vi "TAT_Varient Creater.vi"(8 "error in (no error)":errorcluster) -> (0 "error out":errorcluster)   [LabVIEW 2017]
uses:
  <vilib>/Utility/miscctls.llb/LVRangeTypeDef.ctl
  <vilib>/addons/database/Connection.llb/Conn ObjectReference.ctl
  <vilib>/Utility/miscctls.llb/LVRowAndColumnUnsignedTypeDef.ctl
  b1939813-2d0c-4b6e-8ee7-2e1edd5edc28.vi
  <vilib>/Utility/config.llb/Read Key (I32).vi
  <vilib>/Utility/config.llb/Read Key (String).vi
  <vilib>/Utility/config.llb/Read Key (Boolean).vi
  <vilib>/Utility/config.llb/Write Key (U32).vi
  <vilib>/Utility/config.llb/Write Key (String).vi
  <vilib>/Utility/config.llb/Write Key (Boolean).vi
  <vilib>/Utility/config.llb/NI_LVConfig.lvlib
  <vilib>/addons/database/NI_Database_API.lvlib
panel:
  in  "HARNESS CODE":string
  in  "STATION 2\nBYPASS":bool
  in  "Vertical Slider Control":dbl(slide)=1.0 scale=1.0..-1.0
  in  "CANCLE 3":bool
  in  "PRINTING":bool
  in  "Manual print":bool
  in  "Cancle 2":bool
  in  "Delete Button":bool
  in  "Cancle":bool
  in  "Save Button":bool
  in  "TORISHI CODE":string
  in  "PART NUMBER":string
  in  "Delete Square":bool
  in  "EDIT & SAVE":bool
  out "Varient Details":string[][](table)
  in  "BATCH SIZE":u16=1 min=1 max=100 step=1
  in  "VARIENT NUMBER":u16=1 min=1 max=100 step=1
  in  "HOME":bool
  in  "UPDATE TABLE":bool
  in  "PART NAME":string(combo)
  # "Varient Creater Station 1"
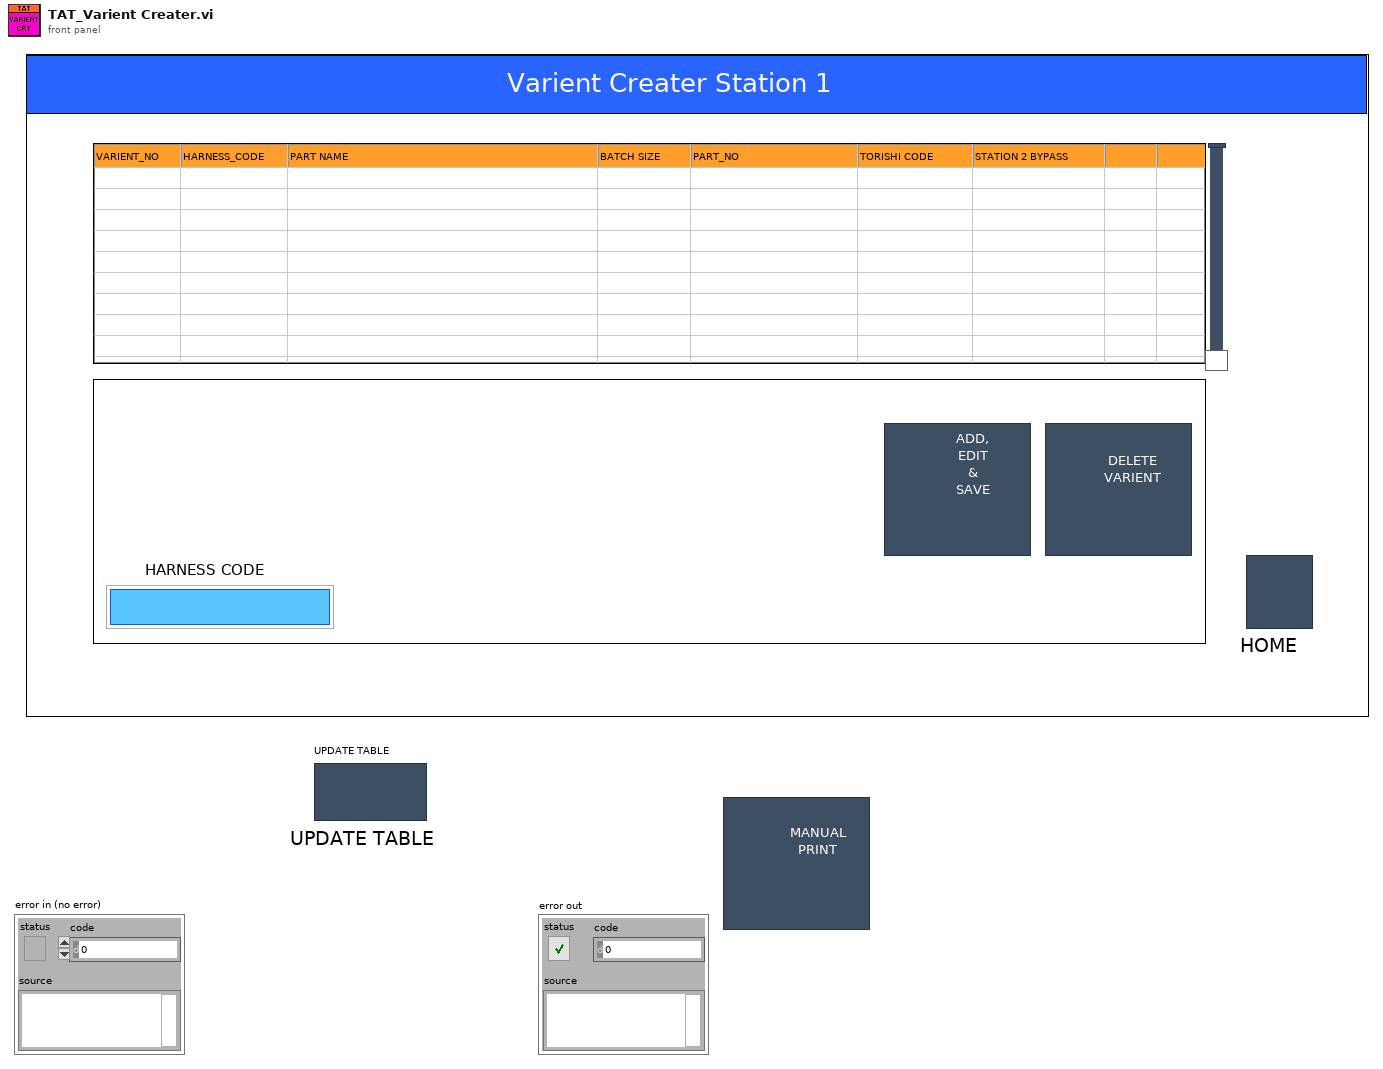
[diagram p1: front panel]
types:
  T1 = enum8{"Enabled", "Disabled", "Disabled and Grayed Out"}
  T2 = enum32{"invalid app kind", "Development System", "Run Time System", "Student Edition", "Embedded LabVIEW", "Evaluation", "Custom"}
  T3 = typedef "NI_LVConfig.lvlib/Config Data RefNum.ctl" = refnum<k1>
  T4 = typedef "LVRangeTypeDef.ctl" = cluster{"Minimum":dbl, "Maximum":dbl, "Increment":dbl, "Minor Increment":dbl, "Start":dbl}
  T5 = typedef "NI_Database_API.lvlib/Conn ObjectReference.ctl" = refnum<k1>
  T6 = cluster{"Varient number":u16, "Part name":string, "connection reference":T5, "Batch_Size":u16, "PART_NO":string, "TORISHI_CODE":string, "scanner com":refnum<visa-resource-name>, "Part Name List":string[], "Varient path":path, "Current Varient path":path, "Communication path":path, "Package path":path, "Part PRN path":path, "Station2 printer IP":string, "Station1 printer IP":string, "Current Serial Number":string, "Station1_QR":string, "Serial_Number":path, "PRIVIOUS code":string[], "Barcode station2 log":string, "Barcode station2 Up":string, "HARNESS CODE":string, "Station 1 bypass":bool}
  T7 = typedef "LVRowAndColumnUnsignedTypeDef.ctl" = cluster{"Row":u32, "Column":u32}
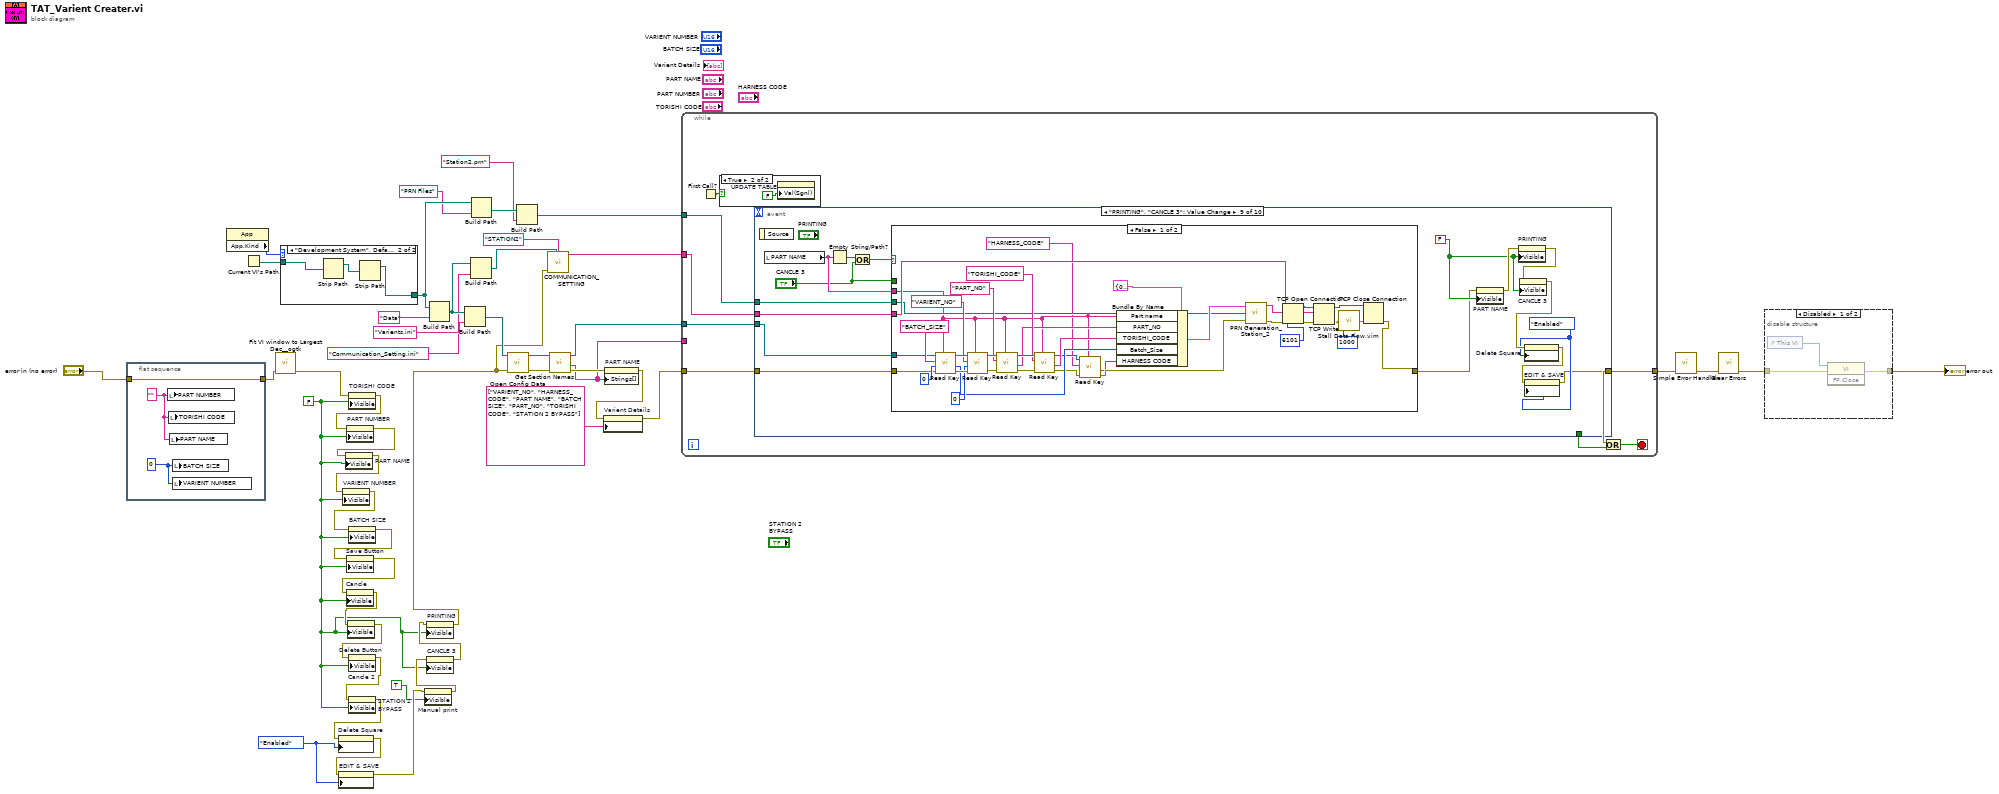
[diagram p0: block diagram]
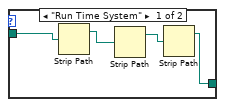
[diagram p3: hidden frame]
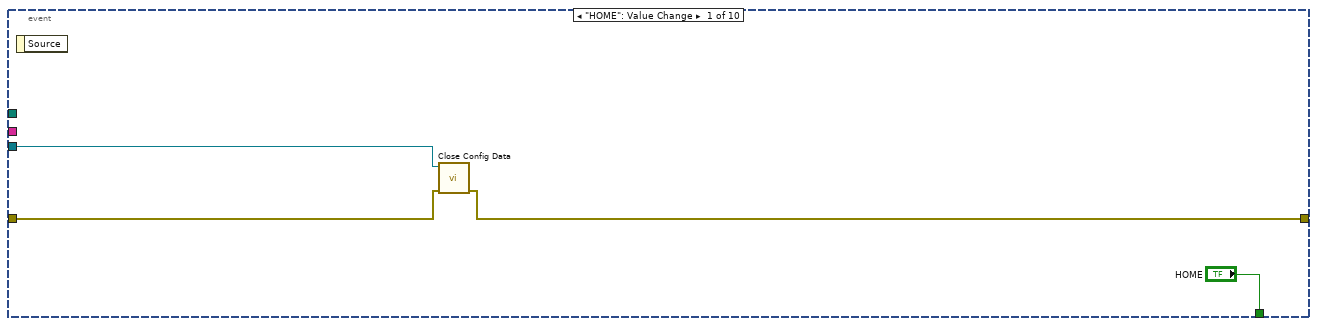
[diagram p5: hidden frame]
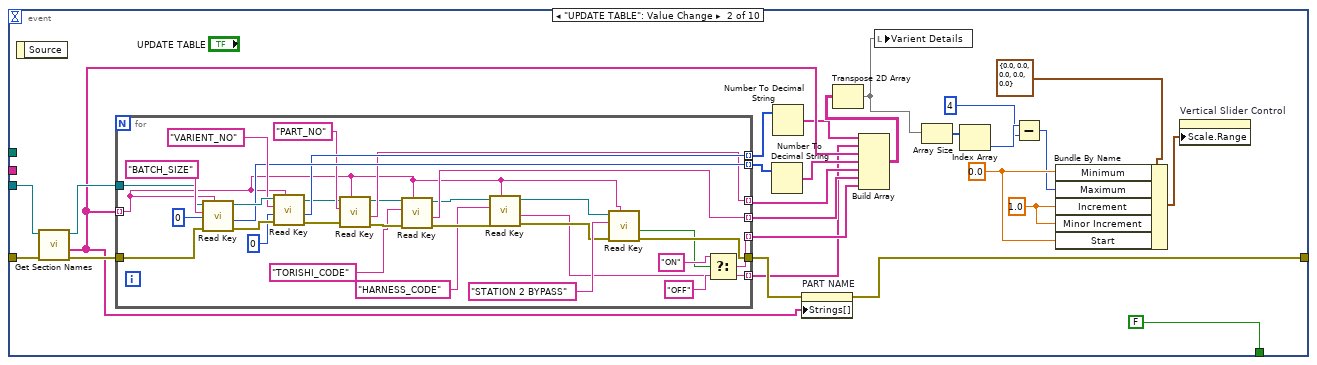
[diagram p6: hidden frame]
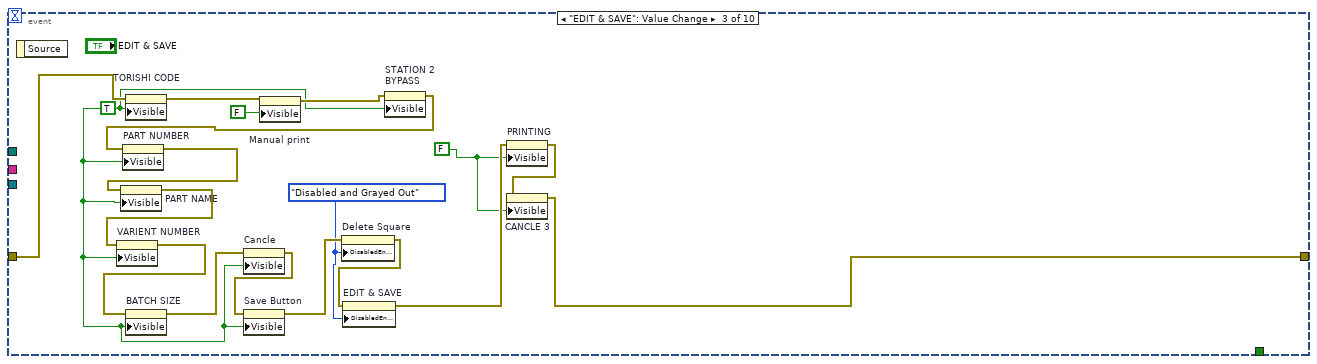
[diagram p7: hidden frame]
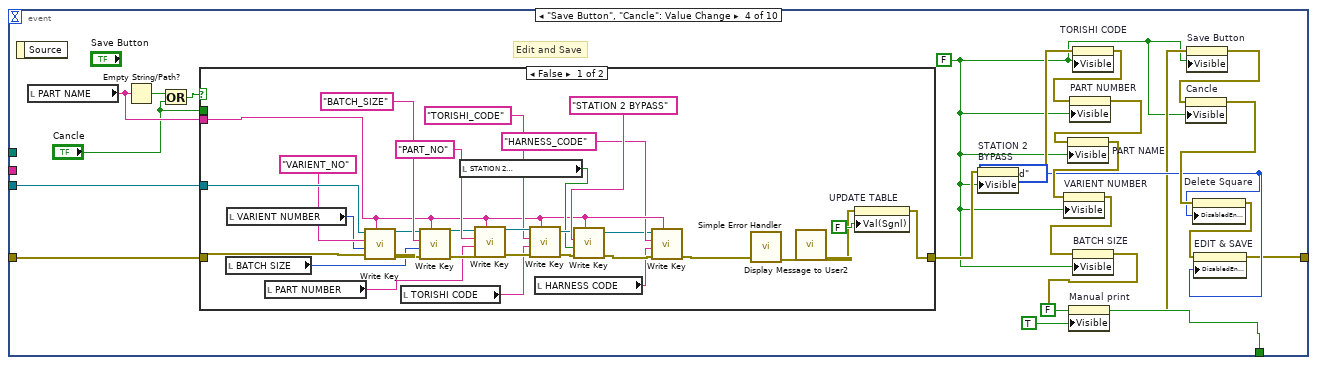
[diagram p8: hidden frame]
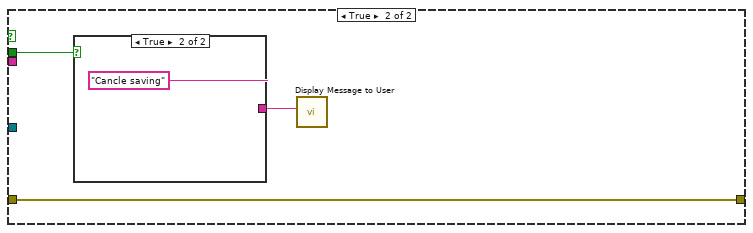
[diagram p9: hidden frame]
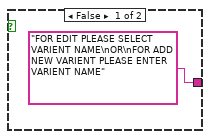
[diagram p10: hidden frame]
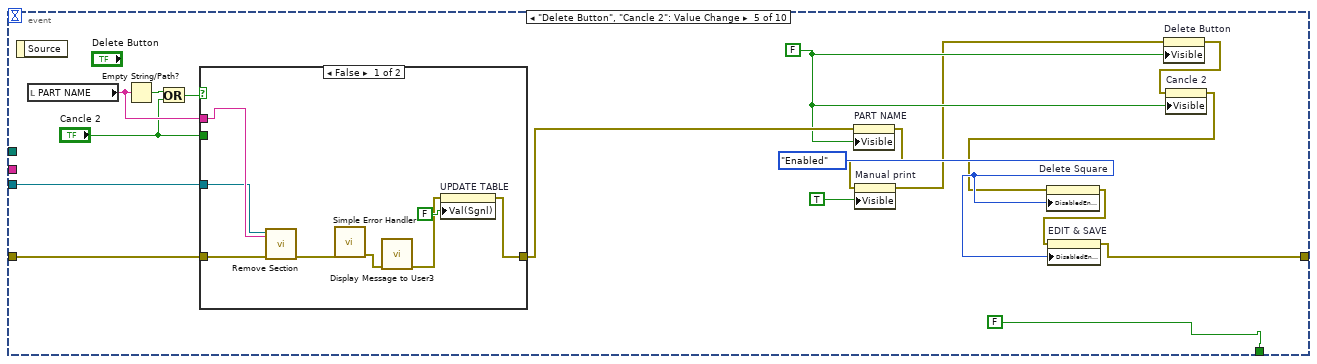
[diagram p11: hidden frame]
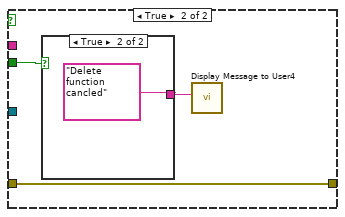
[diagram p12: hidden frame]
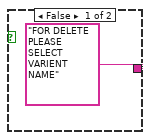
[diagram p13: hidden frame]
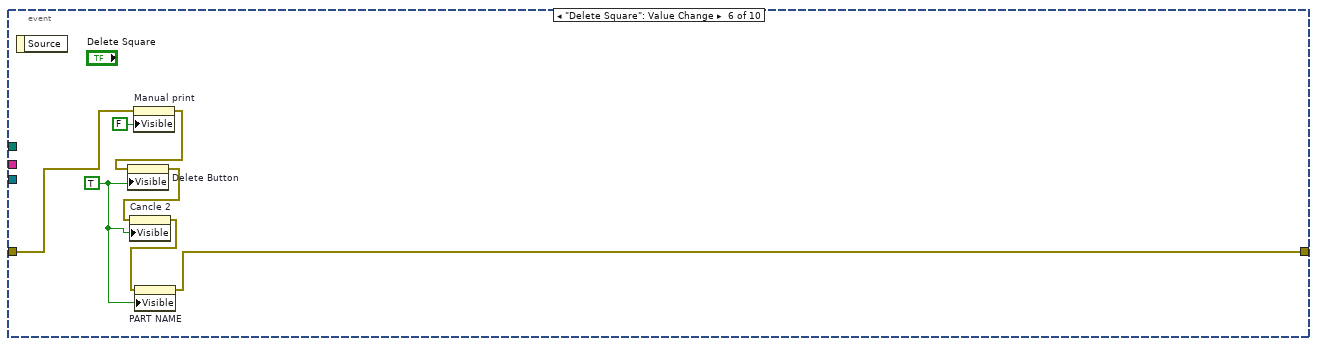
[diagram p14: hidden frame]
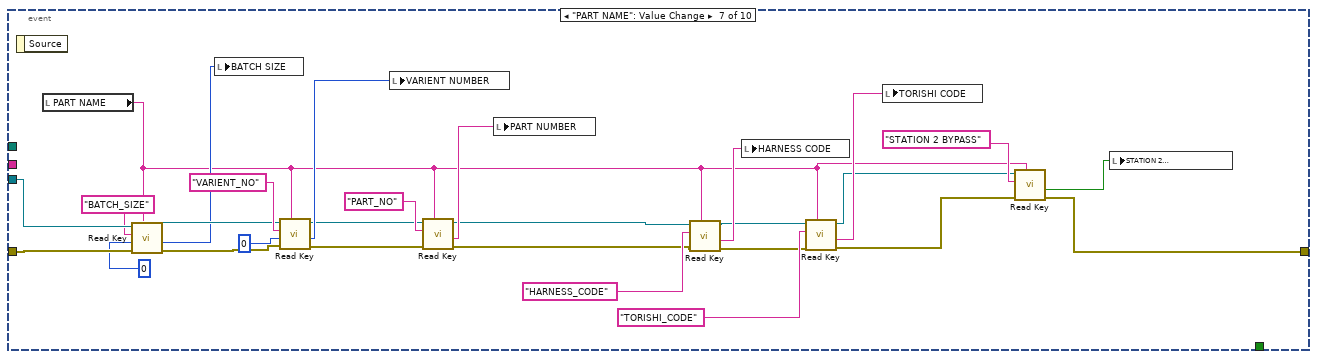
[diagram p15: hidden frame]
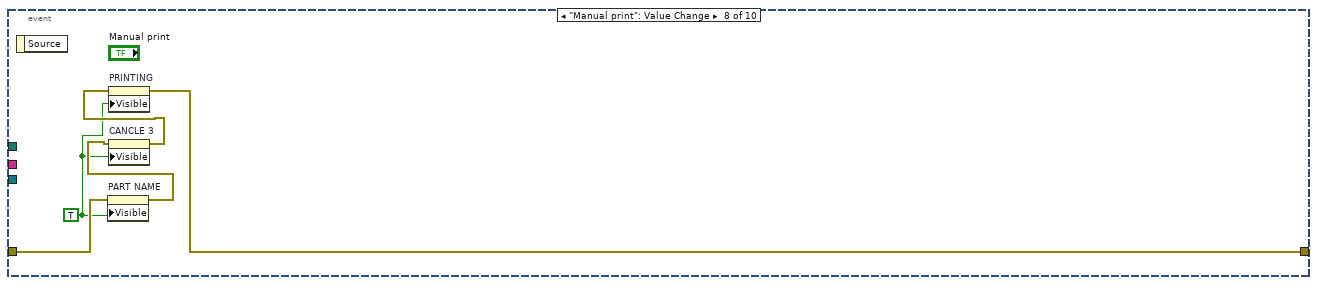
[diagram p16: hidden frame]
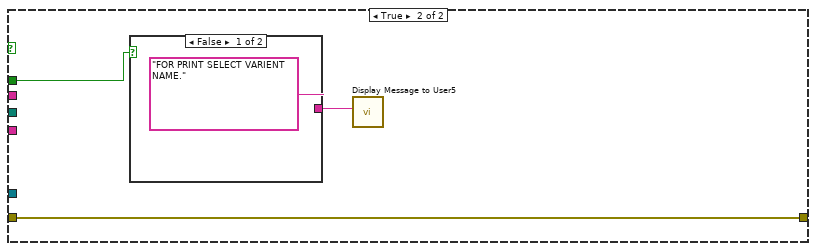
[diagram p17: hidden frame]
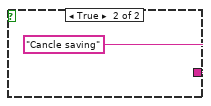
[diagram p18: hidden frame]
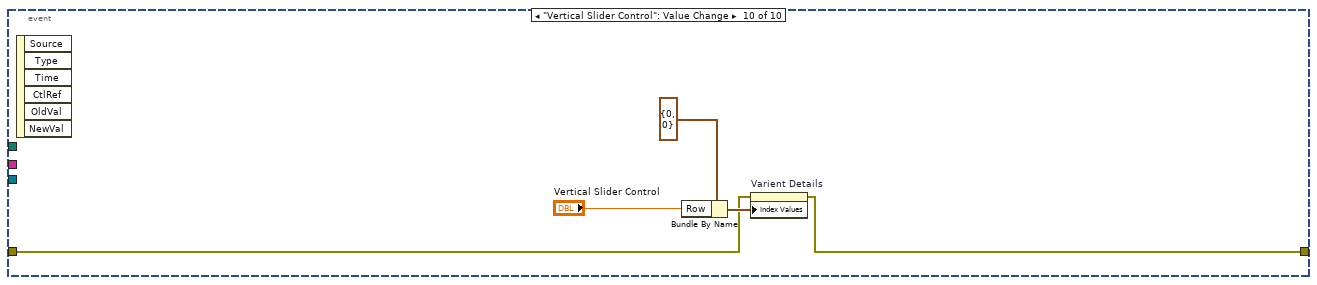
[diagram p19: hidden frame]
diagram:
  w22 = T1."Enabled" ("Disabled")
  w3 = FALSE
  n1 = flat-sequence {
    tunnel: [w49] -> w30
    tunnel: "error in (no error)" -> [w49]
    frame #0 {
      w50 = u16 0 ("BATCH SIZE")
      w51 = "" ("PART NUMBER")
      n2 = local write "PART NUMBER"(w51) -> ()
      n3 = local write "TORISHI CODE"(w51) -> ()
      n4 = local write "PART NAME"(w51) -> ()
      n5 = local write "BATCH SIZE"(w50) -> ()
      n6 = local write "VARIENT NUMBER"(w50) -> ()
    }
  }
  n7 = property class="App"() -> ("App.Kind"=w43:T2)  [unwired: 2 in, 2 out]
  n8 = Current VI's Path() -> (path=w44:path)
  n9 = call <userlib>:"Fit VI window to Largest Dec__ogtk.vi"("error in (no error)"=w30) -> ("error out"=w25:errorcluster)  [unwired: 5 in, 1 out]
  n10 = case shown="\"Development System\", Default" w43 {
    tunnel: w44 -> [w53 w57]
    tunnel: [w52 w56] -> w8
    frame "Run Time System" {
      n11 = Strip Path(path=w53) -> (stripped path=w55:path)  [unwired: 1 out]
      n12 = Strip Path(path=w55) -> (stripped path=w54:path)  [unwired: 1 out]
      n13 = Strip Path(path=w54) -> (stripped path=w52:path)  [unwired: 1 out]
    }
    frame "Development System", Default {
      n14 = Strip Path(path=w57) -> (stripped path=w58:path)  [unwired: 1 out]
      n15 = Strip Path(path=w58) -> (stripped path=w56:path)  [unwired: 1 out]
    }
  }
  n16 = property on="TORISHI CODE" class="Str"(error in=w25, "Visible"=w3) -> (error out=w29:errorcluster)  [unwired: 1 in, 1 out]
  n17 = property on="PART NUMBER" class="Str"(error in=w29, "Visible"=w3) -> (error out=w28:errorcluster)  [unwired: 1 in, 1 out]
  n18 = property on="PART NAME" class="CmbBox"(error in=w28, "Visible"=w3) -> (error out=w27:errorcluster)  [unwired: 1 in, 1 out]
  n19 = property on="VARIENT NUMBER" class="DigNum (strict)"(error in=w27, "Visible"=w3) -> (error out=w26:errorcluster)  [unwired: 1 in, 1 out]
  n20 = property on="BATCH SIZE" class="DigNum (strict)"(error in=w26, "Visible"=w3) -> (error out=w24:errorcluster)  [unwired: 1 in, 1 out]
  n21 = property on="Save Button" class="Bool"(error in=w24, "Visible"=w3) -> (error out=w21:errorcluster)  [unwired: 1 in, 1 out]
  n22 = property on="Cancle" class="Bool"(error in=w21, "Visible"=w3) -> (error out=w20:errorcluster)  [unwired: 1 in, 1 out]
  n23 = property on="Delete Button" class="Bool"(error in=w20, "Visible"=w3) -> (error out=w19:errorcluster)  [unwired: 1 in, 1 out]
  n24 = property on="Cancle 2" class="Bool"(error in=w19, "Visible"=w3) -> (error out=w2:errorcluster)  [unwired: 1 in, 1 out]
  n25 = property on="STATION 2\nBYPASS" class="Bool (strict)"(error in=w2, "Visible"=w3) -> (error out=w1:errorcluster)  [unwired: 1 in, 1 out]
  n26 = property on="Delete Square" class="Bool"(error in=w1, "DisabledEnum"=w22) -> (error out=w23:errorcluster)  [unwired: 1 in, 1 out]
  n27 = property on="EDIT & SAVE" class="Bool"(error in=w23, "DisabledEnum"=w22) -> (error out=w17:errorcluster)  [unwired: 1 in, 1 out]
  n28 = property on="Manual print" class="Bool"(error in=w17, "Visible"=TRUE) -> (error out=w16:errorcluster)  [unwired: 1 in, 1 out]
  n29 = property on="CANCLE 3" class="Bool"(error in=w16, "Visible"=w3) -> (error out=w18:errorcluster)  [unwired: 1 in, 1 out]
  n30 = property on="PRINTING" class="Bool"(error in=w18, "Visible"=w3) -> (error out=w10:errorcluster)  [unwired: 1 in, 1 out]
  n31 = Build Path(base path=w8, name or relative path="Data") -> (appended path=w14:path)
  n32 = Build Path(base path=w14, name or relative path="Varients.ini") -> (appended path=w42:path)
  n33 = Build Path(base path=w14, name or relative path="Communication_Setting.ini") -> (appended path=w11:path)
  n34 = Build Path(base path=w8, name or relative path="PRN Files") -> (appended path=w6:path)
  n35 = call <vilib>:"Open Config Data.vi"("error in (no error)"=w10, "configuration file path"=w42) -> ("error out"=w38:errorcluster, "refnum"=w39:T3)  [unwired: 7 in, 1 out]
  n36 = Build Path(base path=w6, name or relative path="Station2.prn") -> (appended path=w4:path)
  n37 = call "COMMUNICATION_SETTING.vi"("communication path"=w11, "error in"=w10, "STATION"="STATION2") -> ("PRINT_COM"=w9:string)  [unwired: 6 in, 2 out]
  n38 = call <vilib>:"Get Section Names.vi"("error in (no error)"=w38, "refnum"=w39) -> ("error out"=w37:errorcluster, "section names"=w32:string[], "refnum out"=w36:T3)  [unwired: 7 in]
  n39 = property on="PART NAME" class="CmbBox"(error in=w37, "Strings[]"=w32) -> (error out=w35:errorcluster)  [unwired: 1 in, 1 out]
  n40 = property on="Varient Details" class="Tbl (strict)"(error in=w35, "Column Headers[]"=string[] ["VARIENT_NO", "HARNESS_CODE", "PART NAME", "BATCH SIZE", "PART_NO", "TORISHI CODE", "STATION 2 BYPASS"] ("Column Header Strings[]")) -> (error out=w34:errorcluster)  [unwired: 1 in, 1 out]
  n41 = while {
    tunnel: w34 -> [w65]
    tunnel: [w63] -> w45
    tunnel: w36 -> [w62]
    tunnel: w32 -> [_]
    tunnel: w9 -> [w60]
    tunnel: w4 -> [w59]
    stop <- w64 stop-if-true
    n42 = First Call?() -> (First Call?: T/F=w61:bool)
    n43 = case shown="True" w61 {
      frame False {
      }
      frame True {
        n44 = property on="UPDATE TABLE" class="Bool (strict)"("Val(Sgnl)"=FALSE) -> ()  [unwired: 2 in, 2 out]
      }
    }
    n45 = event shown="[8] \"PRINTING\", \"CANCLE 3\": Value Change" {
      selector: _ -> [_ _ _ _ _ _ _ _ _ _]
      dyn-events: _ -> [_ _ _ _ _ _ _ _ _ _]
      timeout: _ -> [_ _ _ _ _ _ _ _ _ _]
      tunnel: ["HOME" FALSE ("stop") _ FALSE ("stop") FALSE ("stop") _ _ _ _ _] -> w66
      tunnel: w65 -> [w70 w92 w143 w166 w218 w235 w268 w271 w289 w332]
      tunnel: [w69 w84 w133 w153 w210 w238 w251 w270 w278 w333] -> w63
      tunnel: w62 -> [w68 w90 _ w167 w219 _ w267 _ w285 _]
      tunnel: w60 -> [_ _ _ _ _ _ _ _ w276 _]
      tunnel: w59 -> [_ _ _ _ _ _ _ _ w275 _]
      event "HOME": Value Change {
        n46 = event-data() -> ()  [unwired: 1 in, 1 out]
        n47 = call <vilib>:"Close Config Data.vi"("error in (no error)"=w70, "refnum"=w68) -> ("error out"=w69:errorcluster)  [unwired: 8 in, 1 out]
      }
      event "UPDATE TABLE": Value Change {
        w81 = 1.0 ("Increment")
        w80 = 0.0 ("Minimum")
        n48 = event-data() -> ()  [unwired: 1 in, 1 out]
        n49 = call <vilib>:"Get Section Names.vi"("error in (no error)"=w92, "refnum"=w90) -> ("error out"=w91:errorcluster, "section names"=w85:string[], "refnum out"=w89:T3)  [unwired: 7 in]
        n50 = for {
          tunnel: [w110] -> w86
          tunnel: w91 -> [w122]
          tunnel: w85 -> [w102] mode=indexing
          tunnel: w89 -> [w121]
          tunnel: [w120] -> w95 mode=indexing
          tunnel: [w119] -> w96 mode=indexing
          tunnel: [w115] -> w88 mode=indexing
          tunnel: [w111] -> w87 mode=indexing
          tunnel: [w105] -> w74 mode=indexing
          tunnel: [w98] -> w72 mode=indexing
          n51 = call-poly <vilib>:"Read Key.vi"("section"=w102, "error in (no error)"=w122, "default value"=0, "key"="BATCH_SIZE", "refnum"=w121) -> ("error out"=w128:errorcluster, "value"=w120:i32, "refnum out"=w127:T3)  [unwired: 3 in, 1 out]
          n52 = call-poly <vilib>:"Read Key.vi"("section"=w102, "error in (no error)"=w128, "default value"=0, "key"="VARIENT_NO", "refnum"=w127) -> ("error out"=w118:errorcluster, "value"=w119:i32, "refnum out"=w116:T3)  [unwired: 3 in, 1 out]
          n53 = call-poly <vilib>:"Read Key.vi"("section"=w102, "error in (no error)"=w118, "key"="PART_NO", "refnum"=w116) -> ("error out"=w114:errorcluster, "value"=w115:string, "refnum out"=w113:T3)  [unwired: 4 in, 1 out]
          n54 = call-poly <vilib>:"Read Key.vi"("section"=w102, "error in (no error)"=w114, "key"="TORISHI_CODE", "refnum"=w113) -> ("error out"=w101:errorcluster, "value"=w111:string, "refnum out"=w104:T3)  [unwired: 4 in, 1 out]
          n55 = call-poly <vilib>:"Read Key.vi"("section"=w102, "error in (no error)"=w101, "key"="HARNESS_CODE", "refnum"=w104) -> ("error out"=w100:errorcluster, "value"=w98:string, "refnum out"=w103:T3)  [unwired: 4 in, 1 out]
          n56 = call-poly <vilib>:"Read Key.vi"("section"=w102, "error in (no error)"=w100, "key"="STATION 2 BYPASS", "refnum"=w103) -> ("error out"=w110:errorcluster, "value"=w106:bool)  [unwired: 4 in, 2 out]
          n57 = Select(t="ON" ("String"), s=w106, f="OFF" ("String")) -> (s? t:f=w105:string)
        }
        n58 = Number To Decimal String(number=w95) -> (decimal integer string=w94:string[])  [unwired: 1 in]
        n59 = Number To Decimal String(number=w96) -> (decimal integer string=w73:string[])  [unwired: 1 in]
        n60 = property on="PART NAME" class="CmbBox"(error in=w86, "Strings[]"=w85) -> (error out=w84:errorcluster)  [unwired: 1 in, 1 out]
        n61 = Build Array(w73, w72, w85, w94, w88, w87, w74) -> (w93:string[][])
        n62 = Transpose 2D Array(2D array=w93) -> (transposed array=w83:string[][])
        n63 = local write "Varient Details"(w83) -> ()
        n64 = Array Size(array=w83) -> (size(s)=w82:i32[])
        n65 = Index Array(array=w82) -> (element=w77:i32)  [unwired: 1 in]
        n66 = Subtract(x=w77, y=4) -> (x-y=w76:i32)
        n67 = Bundle By Name(cluster=T4 {"Minimum"=0.0, "Maximum"=0.0, "Increment"=0.0, "Minor Increment"=0.0, "Start"=0.0} ("Scale.Range"), "Minimum"=w80, "Maximum"=w76, "Increment"=w81, "Minor Increment"=w81, "Start"=w80) -> (w79:T4)
        n68 = property on="Vertical Slider Control" class="Slide (strict)"("Scale.Range"=w79) -> ()  [unwired: 2 in, 2 out]
      }
      event "EDIT & SAVE": Value Change {
        w132 = FALSE
        w140 = T1."Disabled and Grayed Out" ("Disabled")
        w129 = TRUE
        n69 = event-data() -> ()  [unwired: 1 in, 1 out]
        n70 = property on="TORISHI CODE" class="Str"(error in=w143, "Visible"=w129) -> (error out=w137:errorcluster)  [unwired: 1 in, 1 out]
        n71 = property on="Manual print" class="Bool"(error in=w137, "Visible"=FALSE) -> (error out=w131:errorcluster)  [unwired: 1 in, 1 out]
        n72 = property on="STATION 2\nBYPASS" class="Bool (strict)"(error in=w131, "Visible"=w129) -> (error out=w130:errorcluster)  [unwired: 1 in, 1 out]
        n73 = property on="PART NUMBER" class="Str"(error in=w130, "Visible"=w129) -> (error out=w144:errorcluster)  [unwired: 1 in, 1 out]
        n74 = property on="PART NAME" class="CmbBox"(error in=w144, "Visible"=w129) -> (error out=w145:errorcluster)  [unwired: 1 in, 1 out]
        n75 = property on="VARIENT NUMBER" class="DigNum (strict)"(error in=w145, "Visible"=w129) -> (error out=w146:errorcluster)  [unwired: 1 in, 1 out]
        n76 = property on="BATCH SIZE" class="DigNum (strict)"(error in=w146, "Visible"=w129) -> (error out=w138:errorcluster)  [unwired: 1 in, 1 out]
        n77 = property on="Cancle" class="Bool"(error in=w138, "Visible"=w129) -> (error out=w139:errorcluster)  [unwired: 1 in, 1 out]
        n78 = property on="Save Button" class="Bool"(error in=w139, "Visible"=w129) -> (error out=w142:errorcluster)  [unwired: 1 in, 1 out]
        n79 = property on="Delete Square" class="Bool"(error in=w142, "DisabledEnum"=w140) -> (error out=w141:errorcluster)  [unwired: 1 in, 1 out]
        n80 = property on="EDIT & SAVE" class="Bool"(error in=w141, "DisabledEnum"=w140) -> (error out=w134:errorcluster)  [unwired: 1 in, 1 out]
        n81 = property on="PRINTING" class="Bool"(error in=w134, "Visible"=w132) -> (error out=w135:errorcluster)  [unwired: 1 in, 1 out]
        n82 = property on="CANCLE 3" class="Bool"(error in=w135, "Visible"=w132) -> (error out=w133:errorcluster)  [unwired: 1 in, 1 out]
      }
      event "Save Button", "Cancle": Value Change {
        w154 = T1."Enabled" ("Disabled")
        w147 = FALSE
        # "Edit and Save"
        n83 = event-data() -> ()  [unwired: 1 in, 1 out]
        n84 = local read "PART NAME"() -> (w165:string)
        n85 = Empty String/Path?(string/path=w165) -> (empty?=w164:bool)
        n86 = Or(x=w164, y="Cancle") -> (x .or. y?=w163:bool)
        n87 = case shown="False" w163 {
          tunnel: w166 -> [w197 w201]
          tunnel: [w191 w201] -> w149
          tunnel: w167 -> [w195 _]
          tunnel: w165 -> [w174 _]
          tunnel: "Cancle" -> [_ w199]
          frame False {
            n88 = local read "BATCH SIZE"() -> (w190:u16)
            n89 = local read "VARIENT NUMBER"() -> (w189:u16)
            n90 = local read "PART NUMBER"() -> (w179:string)
            n91 = call-poly <vilib>:"Write Key.vi"("section"=w174, "error in (no error)"=w197, "value"=w189, "key"="VARIENT_NO", "refnum"=w195) -> ("error out"=w196:errorcluster, "refnum out"=w194:T3)  [unwired: 4 in, 1 out]
            n92 = local read "TORISHI CODE"() -> (w180:string)
            n93 = call-poly <vilib>:"Write Key.vi"("section"=w174, "error in (no error)"=w196, "value"=w190, "key"="BATCH_SIZE", "refnum"=w194) -> ("error out"=w184:errorcluster, "refnum out"=w182:T3)  [unwired: 4 in, 1 out]
            n94 = local read "STATION 2\nBYPASS"() -> (w175:bool)
            n95 = call-poly <vilib>:"Write Key.vi"("section"=w174, "error in (no error)"=w184, "value"=w179, "key"="PART_NO", "refnum"=w182) -> ("error out"=w185:errorcluster, "refnum out"=w186:T3)  [unwired: 4 in, 1 out]
            n96 = call-poly <vilib>:"Write Key.vi"("section"=w174, "error in (no error)"=w185, "value"=w180, "key"="TORISHI_CODE", "refnum"=w186) -> ("error out"=w177:errorcluster, "refnum out"=w176:T3)  [unwired: 4 in, 1 out]
            n97 = local read "HARNESS CODE"() -> (w169:string)
            n98 = call-poly <vilib>:"Write Key.vi"("section"=w174, "error in (no error)"=w177, "value"=w175, "key"="STATION 2 BYPASS", "refnum"=w176) -> ("error out"=w173:errorcluster, "refnum out"=w170:T3)  [unwired: 4 in, 1 out]
            n99 = call-poly <vilib>:"Write Key.vi"("section"=w174, "error in (no error)"=w173, "value"=w169, "key"="HARNESS_CODE", "refnum"=w170) -> ("error out"=w172:errorcluster)  [unwired: 4 in, 2 out]
            n100 = call <vilib>:"Simple Error Handler.vi"("error in (no error)"=w172) -> ("error out"=w188:errorcluster)  [unwired: 4 in, 4 out]
            n101 = call "Display Message to User2"("error in (no error)"=w188) -> ("error out"=w187:errorcluster)  [unwired: 9 in, 1 out]
            n102 = property on="UPDATE TABLE" class="Bool (strict)"(error in=w187, "Val(Sgnl)"=FALSE) -> (error out=w191:errorcluster)  [unwired: 1 in, 1 out]
          }
          frame True {
            n103 = case shown="True" w199 {
              tunnel: ["FOR EDIT PLEASE SELECT VARIENT NAME\nOR\nFOR ADD NEW VARIENT PLEASE ENTER VARIENT NAME" "Cancle saving"] -> w200
              frame False {
              }
              frame True {
              }
            }
            n104 = call "Display Message to User"("Message"=w200) -> ()  [unwired: 9 in, 2 out]
          }
        }
        n105 = property on="STATION 2\nBYPASS" class="Bool (strict)"(error in=w149, "Visible"=w147) -> (error out=w148:errorcluster)  [unwired: 1 in, 1 out]
        n106 = property on="TORISHI CODE" class="Str"(error in=w148, "Visible"=w147) -> (error out=w161:errorcluster)  [unwired: 1 in, 1 out]
        n107 = property on="PART NUMBER" class="Str"(error in=w161, "Visible"=w147) -> (error out=w160:errorcluster)  [unwired: 1 in, 1 out]
        n108 = property on="PART NAME" class="CmbBox"(error in=w160, "Visible"=w147) -> (error out=w159:errorcluster)  [unwired: 1 in, 1 out]
        n109 = property on="VARIENT NUMBER" class="DigNum (strict)"(error in=w159, "Visible"=w147) -> (error out=w158:errorcluster)  [unwired: 1 in, 1 out]
        n110 = property on="BATCH SIZE" class="DigNum (strict)"(error in=w158, "Visible"=w147) -> (error out=w151:errorcluster)  [unwired: 1 in, 1 out]
        n111 = property on="Manual print" class="Bool"(error in=w151, "Visible"=TRUE) -> (error out=w150:errorcluster)  [unwired: 1 in, 1 out]
        n112 = property on="Save Button" class="Bool"(error in=w150, "Visible"=w147) -> (error out=w156:errorcluster)  [unwired: 1 in, 1 out]
        n113 = property on="Cancle" class="Bool"(error in=w156, "Visible"=w147) -> (error out=w155:errorcluster)  [unwired: 1 in, 1 out]
        n114 = property on="Delete Square" class="Bool"(error in=w155, "DisabledEnum"=w154) -> (error out=w157:errorcluster)  [unwired: 1 in, 1 out]
        n115 = property on="EDIT & SAVE" class="Bool"(error in=w157, "DisabledEnum"=w154) -> (error out=w153:errorcluster)  [unwired: 1 in, 1 out]
      }
      event "Delete Button", "Cancle 2": Value Change {
        w212 = T1."Enabled" ("Disabled")
        w207 = FALSE
        n116 = event-data() -> ()  [unwired: 1 in, 1 out]
        n117 = local read "PART NAME"() -> (w217:string)
        n118 = Empty String/Path?(string/path=w217) -> (empty?=w216:bool)
        n119 = Or(x=w216, y="Cancle 2") -> (x .or. y?=w215:bool)
        n120 = case shown="False" w215 {
          tunnel: w218 -> [w222 w231]
          tunnel: [w227 w231] -> w211
          tunnel: w219 -> [w223 _]
          tunnel: w217 -> [w224 _]
          tunnel: "Cancle 2" -> [_ w230]
          frame False {
            n121 = call <vilib>:"Remove Section.vi"("section"=w224, "error in (no error)"=w222, "refnum"=w223) -> ("error out"=w221:errorcluster)  [unwired: 6 in, 2 out]
            n122 = call <vilib>:"Simple Error Handler.vi"("error in (no error)"=w221) -> ("error out"=w226:errorcluster)  [unwired: 4 in, 4 out]
            n123 = call "Display Message to User3"("error in (no error)"=w226) -> ("error out"=w225:errorcluster)  [unwired: 9 in, 1 out]
            n124 = property on="UPDATE TABLE" class="Bool (strict)"(error in=w225, "Val(Sgnl)"=FALSE) -> (error out=w227:errorcluster)  [unwired: 1 in, 1 out]
          }
          frame True {
            n125 = case shown="True" w230 {
              tunnel: ["FOR DELETE PLEASE SELECT VARIENT NAME" "Delete function cancled"] -> w229
              frame False {
              }
              frame True {
              }
            }
            n126 = call "Display Message to User4"("Message"=w229) -> ()  [unwired: 9 in, 2 out]
          }
        }
        n127 = property on="PART NAME" class="CmbBox"(error in=w211, "Visible"=w207) -> (error out=w205:errorcluster)  [unwired: 1 in, 1 out]
        n128 = property on="Manual print" class="Bool"(error in=w205, "Visible"=TRUE) -> (error out=w204:errorcluster)  [unwired: 1 in, 1 out]
        n129 = property on="Delete Button" class="Bool"(error in=w204, "Visible"=w207) -> (error out=w209:errorcluster)  [unwired: 1 in, 1 out]
        n130 = property on="Cancle 2" class="Bool"(error in=w209, "Visible"=w207) -> (error out=w208:errorcluster)  [unwired: 1 in, 1 out]
        n131 = property on="Delete Square" class="Bool"(error in=w208, "DisabledEnum"=w212) -> (error out=w213:errorcluster)  [unwired: 1 in, 1 out]
        n132 = property on="EDIT & SAVE" class="Bool"(error in=w213, "DisabledEnum"=w212) -> (error out=w210:errorcluster)  [unwired: 1 in, 1 out]
      }
      event "Delete Square": Value Change {
        w237 = TRUE
        n133 = event-data() -> ()  [unwired: 1 in, 1 out]
        n134 = property on="Manual print" class="Bool"(error in=w235, "Visible"=FALSE) -> (error out=w234:errorcluster)  [unwired: 1 in, 1 out]
        n135 = property on="Delete Button" class="Bool"(error in=w234, "Visible"=w237) -> (error out=w240:errorcluster)  [unwired: 1 in, 1 out]
        n136 = property on="Cancle 2" class="Bool"(error in=w240, "Visible"=w237) -> (error out=w239:errorcluster)  [unwired: 1 in, 1 out]
        n137 = property on="PART NAME" class="CmbBox"(error in=w239, "Visible"=w237) -> (error out=w238:errorcluster)  [unwired: 1 in, 1 out]
      }
      event "PART NAME": Value Change {
        n138 = event-data() -> ()  [unwired: 1 in, 1 out]
        n139 = local read "PART NAME"() -> (w241:string)
        n140 = call-poly <vilib>:"Read Key.vi"("section"=w241, "error in (no error)"=w268, "default value"=0, "key"="BATCH_SIZE", "refnum"=w267) -> ("error out"=w264:errorcluster, "value"=w259:i32, "refnum out"=w263:T3)  [unwired: 3 in, 1 out]
        n141 = local write "BATCH SIZE"(w259) -> ()
        n142 = call-poly <vilib>:"Read Key.vi"("section"=w241, "error in (no error)"=w264, "default value"=0, "key"="VARIENT_NO", "refnum"=w263) -> ("error out"=w258:errorcluster, "value"=w262:i32, "refnum out"=w255:T3)  [unwired: 3 in, 1 out]
        n143 = local write "VARIENT NUMBER"(w262) -> ()
        n144 = call-poly <vilib>:"Read Key.vi"("section"=w241, "error in (no error)"=w258, "key"="PART_NO", "refnum"=w255) -> ("error out"=w245:errorcluster, "value"=w254:string, "refnum out"=w243:T3)  [unwired: 4 in, 1 out]
        n145 = local write "PART NUMBER"(w254) -> ()
        n146 = call-poly <vilib>:"Read Key.vi"("section"=w241, "error in (no error)"=w245, "key"="HARNESS_CODE", "refnum"=w243) -> ("error out"=w244:errorcluster, "value"=w247:string, "refnum out"=w242:T3)  [unwired: 4 in, 1 out]
        n147 = local write "HARNESS CODE"(w247) -> ()
        n148 = call-poly <vilib>:"Read Key.vi"("section"=w241, "error in (no error)"=w244, "key"="TORISHI_CODE", "refnum"=w242) -> ("error out"=w252:errorcluster, "value"=w253:string, "refnum out"=w249:T3)  [unwired: 4 in, 1 out]
        n149 = local write "TORISHI CODE"(w253) -> ()
        n150 = call-poly <vilib>:"Read Key.vi"("section"=w241, "error in (no error)"=w252, "key"="STATION 2 BYPASS", "refnum"=w249) -> ("error out"=w251:errorcluster, "value"=w248:bool)  [unwired: 4 in, 2 out]
        n151 = local write "STATION 2\nBYPASS"(w248) -> ()
      }
      event "Manual print": Value Change {
        w269 = TRUE
        n152 = event-data() -> ()  [unwired: 1 in, 1 out]
        n153 = property on="PART NAME" class="CmbBox"(error in=w271, "Visible"=w269) -> (error out=w273:errorcluster)  [unwired: 1 in, 1 out]
        n154 = property on="CANCLE 3" class="Bool"(error in=w273, "Visible"=w269) -> (error out=w272:errorcluster)  [unwired: 1 in, 1 out]
        n155 = property on="PRINTING" class="Bool"(error in=w272, "Visible"=w269) -> (error out=w270:errorcluster)  [unwired: 1 in, 1 out]
      }
      event "PRINTING", "CANCLE 3": Value Change {
        w279 = T1."Enabled" ("Disabled")
        w280 = FALSE
        n156 = event-data() -> ()  [unwired: 1 in, 1 out]
        n157 = local read "PART NAME"() -> (w286:string)
        n158 = Empty String/Path?(string/path=w286) -> (empty?=w288:bool)
        n159 = Or(x=w288, y="CANCLE 3") -> (x .or. y?=w287:bool)
        n160 = case shown="False" w287 {
          tunnel: w289 -> [w315 w329]
          tunnel: [w306 w329] -> w277
          tunnel: w286 -> [w293 _]
          tunnel: w285 -> [w314 _]
          tunnel: w276 -> [w301 _]
          tunnel: w275 -> [w299 _]
          tunnel: "CANCLE 3" -> [_ w327]
          frame False {
            n161 = call-poly <vilib>:"Read Key.vi"("section"=w293, "error in (no error)"=w315, "default value"=0, "key"="BATCH_SIZE", "refnum"=w314) -> ("error out"=w326:errorcluster, "value"=w304:i32, "refnum out"=w325:T3)  [unwired: 3 in, 1 out]
            n162 = call-poly <vilib>:"Read Key.vi"("section"=w293, "error in (no error)"=w326, "default value"=0, "key"="VARIENT_NO", "refnum"=w325) -> ("error out"=w322:errorcluster, "refnum out"=w321:T3)  [unwired: 3 in, 2 out]
            n163 = call-poly <vilib>:"Read Key.vi"("section"=w293, "error in (no error)"=w322, "key"="PART_NO", "refnum"=w321) -> ("error out"=w323:errorcluster, "value"=w302:string, "refnum out"=w324:T3)  [unwired: 4 in, 1 out]
            n164 = call-poly <vilib>:"Read Key.vi"("section"=w293, "error in (no error)"=w323, "key"="TORISHI_CODE", "refnum"=w324) -> ("error out"=w295:errorcluster, "value"=w305:string, "refnum out"=w294:T3)  [unwired: 4 in, 1 out]
            n165 = call-poly <vilib>:"Read Key.vi"("section"=w293, "error in (no error)"=w295, "key"="HARNESS_CODE", "refnum"=w294) -> ("error out"=w296:errorcluster, "value"=w292:string)  [unwired: 4 in, 2 out]
            n166 = Bundle By Name(cluster=T6 {"Varient number"=0, "Part name"="", "connection reference"=refnum, "Batch_Size"=0, "PART_NO"="", "TORISHI_CODE"="", "scanner com"="", "Part Name List"=[], "Varient path"=path "", "Current Varient path"=path "", "Communication path"=path "", "Package path"=path "", "Part PRN path"=path "", "Station2 printer IP"="", "Station1 printer IP"="", "Current Serial Number"="", "Station1_QR"="", "Serial_Number"=path "", "PRIVIOUS code"=[], "Barcode station2 log"="", "Barcode station2 Up"="", "HARNESS CODE"="", "Station 1 bypass"=FALSE} ("Cluster 2"), "Part name"=w293, "PART_NO"=w302, "TORISHI_CODE"=w305, "Batch_Size"=w304, "HARNESS CODE"=w292) -> (w300:T6)
            n167 = call "PRN Generation_Station_2.vi"("error in (no error)"=w296, "PRN path"=w299, "Cluster"=w300) -> ("error out"=w297:errorcluster, "PRN to Print"=w298:string)  [unwired: 2 in, 2 out]
            n168 = TCP Open Connection(address=w301, remote port or service name=u16 6101, error in (no error)=w297) -> (connection ID=w311:refnum<k5>, error out=w310:errorcluster)  [unwired: 2 in]
            n169 = TCP Write(connection ID=w311, data in=w298, error in (no error)=w310) -> (connection ID out=w313:refnum<k5>, error out=w309:errorcluster)  [unwired: 1 in, 1 out]
            n170 = call "Stall Data Flow.vim"("value in"=w309, "milliseconds to wait"=u32 1000) -> ("value out"=w312:errorcluster)  [unwired: 1 out]
            n171 = TCP Close Connection(connection ID=w313, error in (no error)=w312) -> (error out=w306:errorcluster)  [unwired: 1 in, 1 out]
          }
          frame True {
            n172 = case shown="False" w327 {
              tunnel: ["FOR PRINT SELECT VARIENT NAME." "Cancle saving"] -> w328
              frame False {
              }
              frame True {
              }
            }
            n173 = call "Display Message to User5"("Message"=w328) -> ()  [unwired: 9 in, 2 out]
          }
        }
        n174 = property on="PART NAME" class="CmbBox"(error in=w277, "Visible"=w280) -> (error out=w284:errorcluster)  [unwired: 1 in, 1 out]
        n175 = property on="PRINTING" class="Bool"(error in=w284, "Visible"=w280) -> (error out=w282:errorcluster)  [unwired: 1 in, 1 out]
        n176 = property on="CANCLE 3" class="Bool"(error in=w282, "Visible"=w280) -> (error out=w281:errorcluster)  [unwired: 1 in, 1 out]
        n177 = property on="Delete Square" class="Bool"(error in=w281, "DisabledEnum"=w279) -> (error out=w283:errorcluster)  [unwired: 1 in, 1 out]
        n178 = property on="EDIT & SAVE" class="Bool"(error in=w283, "DisabledEnum"=w279) -> (error out=w278:errorcluster)  [unwired: 1 in, 1 out]
      }
      event "Vertical Slider Control": Value Change {
        n179 = event-data() -> ()  [unwired: 1 in, 6 out]
        n180 = Bundle By Name(cluster=T7 {"Row"=0, "Column"=0} ("Index Values"), "Row"="Vertical Slider Control") -> (w335:T7)
        n181 = property on="Varient Details" class="Tbl (strict)"(error in=w332, "Index Values"=w335) -> (error out=w333:errorcluster)  [unwired: 1 in, 1 out]
      }
    }
    n182 = Or(x=w63, y=w66) -> (x .or. y?=w64:bool)
  }
  n183 = call <vilib>:"Simple Error Handler.vi"("error in (no error)"=w45) -> ("error out"=w48:errorcluster)  [unwired: 4 in, 4 out]
  n184 = call <vilib>:"Clear Errors.vi"("error in (no error)"=w48) -> ("error out"=w47:errorcluster)  [unwired: 5 in, 1 out]
  n185 = disable-structure shown="Disabled" {
    disable-tunnel: w47 -> [w339 w340]
    disable-tunnel: [w338 w340] -> w46
    frame Disabled {
      n186 = control-ref of="This VI"() -> (w337:refnum<vi>)
      n187 = invoke class="VI" method="FP.Close"(reference=w337, error in=w339) -> (error out=w338:errorcluster)  [unwired: 1 in, 2 out]
    }
    frame Enabled {
    }
  }
  "error out" <- w46
